vi "Single Target Field Position.vi"() -> (0 "Goal Found?":bool, 1 "Y":dbl, 3 "X":dbl)   [LabVIEW 2013]
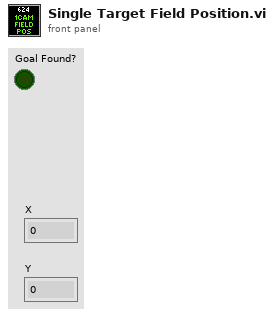
[diagram p1: front panel]
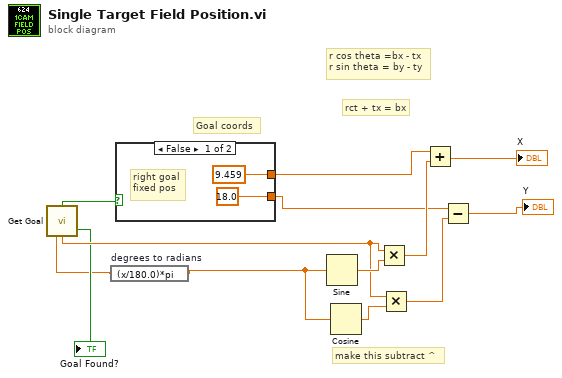
[diagram p0: block diagram]
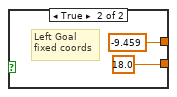
[diagram p2: hidden frame]
diagram:
  # "make this subtract ^"
  # "rct + tx = bx"
  # "r cos theta =bx - tx\nr sin theta = by - ty"
  # "Goal coords"
  n1 = call "Get Goal.vi"() -> ("Left Goal?"=w13:bool, "Field-Rel VisTarget X"=w1:dbl, "Target Distance"=w11:dbl, "Goal Found?"=→"Goal Found?":bool)  [unwired: 7 in, 5 out]
  n2 = expression code="(x/180.0)*pi" "degrees to radians"(w1) -> (w2:dbl)
  n3 = case shown="False" w13 {
    tunnel: [9.459 -9.459] -> w9
    tunnel: [18.0 18.0] -> w4
    frame False {
      # "right goal\nfixed pos"
    }
    frame True {
      # "Left Goal\nfixed coords"
    }
  }
  n4 = Sine(x=w2) -> (sin(x)=w12:dbl)
  n5 = Cosine(x=w2) -> (cos(x)=w10:dbl)
  n6 = Multiply(x=w11, y=w12) -> (x*y=w8:dbl)
  n7 = Multiply(x=w11, y=w10) -> (x*y=w5:dbl)
  n8 = Add(x=w9, y=w8) -> (x+y=→"X":dbl)
  n9 = Subtract(x=w4, y=w5) -> (x-y=→"Y":dbl)
